vi "get_control.vi"(11 "path":string) -> (0 "error out":errorcluster, 3 "control_frontpanel_image":picture)   [LabVIEW 2020]
doc: "Returns a screenshot of the content (frontpanel) of a .ctl file. Use this to understand the content of a LabVIEW type definition or custom control."
uses:
  G-AI Core/G-AI Core.lvlib
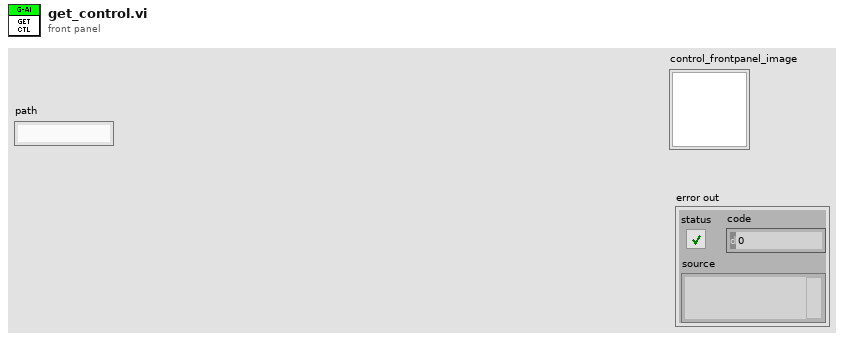
[diagram p1: front panel]
types:
  T1 = typedef "imagedata.ctl" = cluster{"image type":i32, "image depth":i32, "image":u8[], "mask":u8[], "colors":u32[], "Rectangle":cluster{"left":i16, "top":i16, "right":i16, "bottom":i16}}
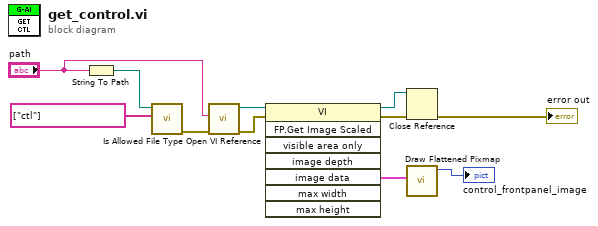
[diagram p0: block diagram]
diagram:
  n1 = String To Path(string="path") -> (path=w3:path)
  n2 = call "Is Allowed File Type.vi"("y"=string[] ["ctl"], "Path"=w3) -> ("error out"=w2:errorcluster)  [unwired: 9 in]
  n3 = call "Open VI Reference.vi"("error in"=w2, "VI Path"="path") -> ("error out"=w9:errorcluster, "VI Refnum"=w10:refnum<vi>)  [unwired: 8 in]
  n4 = invoke class="VI" method="FP.Get Image Scaled"(reference=w10, error in=w9) -> (reference out=w7:refnum<vi>, error out=w8:errorcluster, "image data"=w11:T1)  [unwired: 6 in, 5 out]
  n5 = Close Reference(reference=w7, error in (no error)=w8) -> (error out=→"error out":errorcluster)
  n6 = call <vilib>:"Draw Flattened Pixmap.vi"("image data"=w11) -> ("new picture"=→"control_frontpanel_image":picture)  [unwired: 8 in]
